vi "Keypad Facade.vi"(0 "Data In":T4, 2 "Display State In":T2, 3 "Container State":T3) -> (6 "Data Out":T4, 7 "Display State Out":T2, 8 "Action":T1)   [LabVIEW 2012, in "Keypad.xctl"]
uses:
  Keypad.xctl
  Keypad Data.ctl
  <vilib>/_xctls/Container State.ctl
  Keypad State.ctl
  <vilib>/_xctls/Action.ctl
  <vilib>/_xctls/XControlSupport.lvlib
panel:
  in  "C":bool
  in  "0":bool
  in  "E":bool
  in  "7":bool
  in  "8":bool
  in  "9":bool
  in  "4":bool
  in  "5":bool
  in  "6":bool
  in  "3":bool
  in  "2":bool
  in  "1":bool
  in  "Display":string
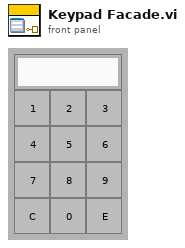
[diagram p1: front panel]
types:
  T1 = typedef "XControlSupport.lvlib/Action.ctl" = cluster{"Data Changed?":bool, "State Changed?":bool, "Action Name":string}
  T2 = typedef "Keypad.xctl/Keypad State.ctl" = cluster{"Current Value":i32}
  T3 = typedef "XControlSupport.lvlib/Container State.ctl" = cluster{"Indicator?":bool, "Run Mode?":bool, " Refnum":refnum<vi>}
  T4 = typedef "Keypad.xctl/Keypad Data.ctl" = i32
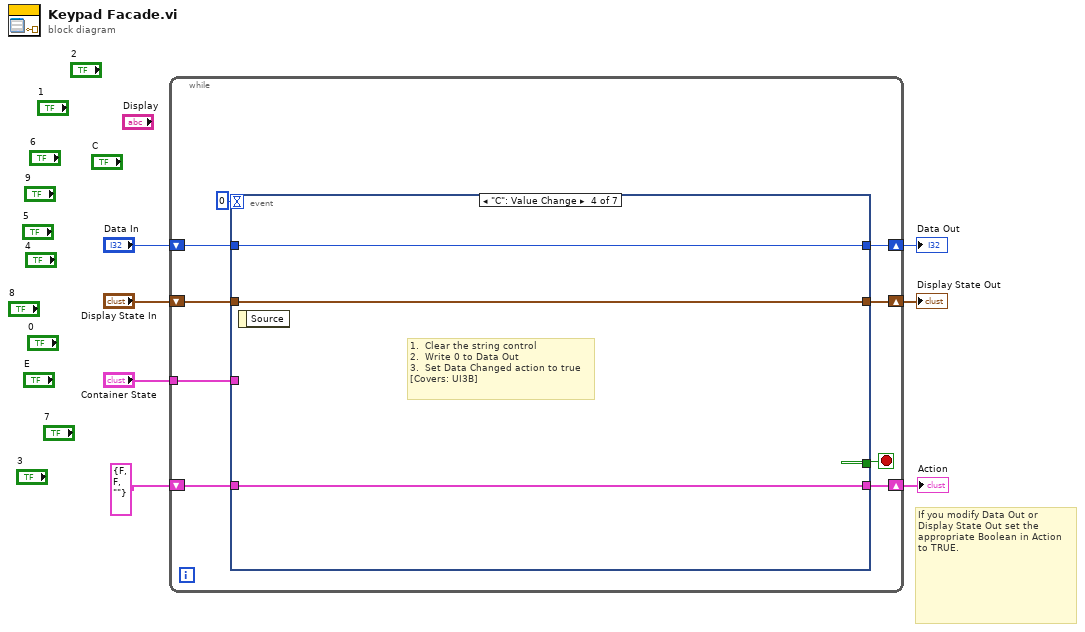
[diagram p0: block diagram]
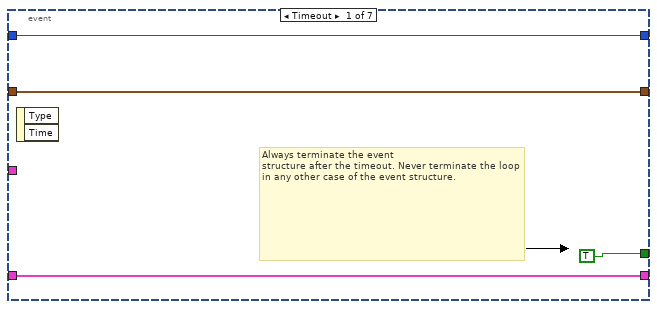
[diagram p2: hidden frame]
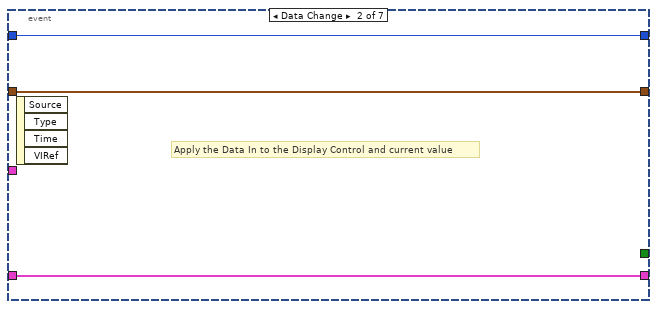
[diagram p3: hidden frame]
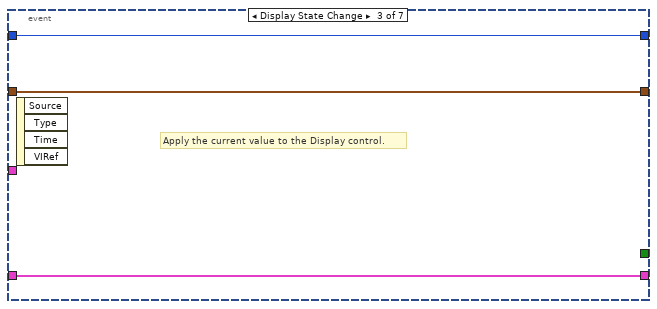
[diagram p4: hidden frame]
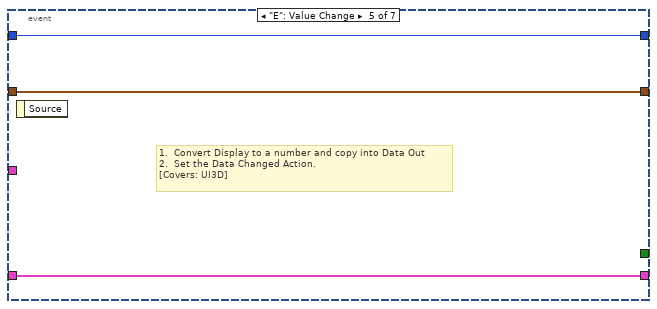
[diagram p5: hidden frame]
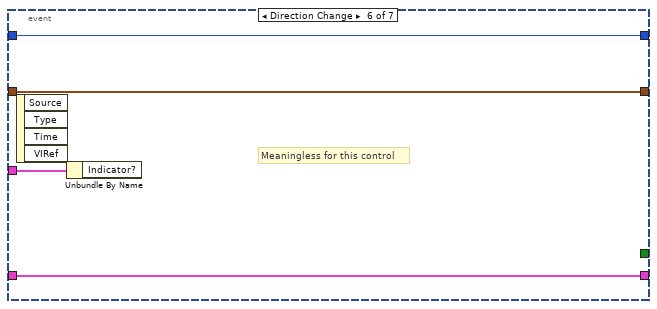
[diagram p6: hidden frame]
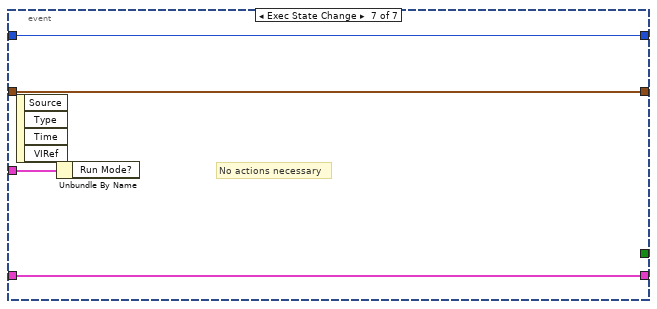
[diagram p7: hidden frame]
diagram:
  # "If you modify Data Out or\nDisplay State Out set the\nappropriate Boolean in Action\nto TRUE."
  n1 = while {
    shift-right: [w15] -> w4
    shift-left: "Display State In" -> [w16]
    tunnel: "Container State" -> [w12]
    shift-right: [w10] -> w7
    shift-left: "Data In" -> [w11]
    shift-right: [w8] -> w2
    shift-left: T1 {"Data Changed?"=FALSE, "State Changed?"=FALSE, "Action Name"=""} ("Action") -> [w9]
    stop <- w14 stop-if-true
    n2 = event shown="[3] \"C\": Value Change" {
      selector: _ -> [_ _ _ _ _ _ _]
      dyn-events: _ -> [_ _ _ _ _ _ _]
      timeout: 0 -> [_ _ _ _ _ _ _]
      tunnel: w16 -> [w18 w22 w26 w28 w31 w35 w39]
      tunnel: [w18 w22 w26 w28 w31 w35 w39] -> w15
      tunnel: [TRUE _ _ _ _ _ _] -> w14
      tunnel: w12 -> [_ _ _ _ _ w36 w40]
      tunnel: w11 -> [w17 w23 w25 w29 w32 w34 w38]
      tunnel: [w17 w23 w25 w29 w32 w34 w38] -> w10
      tunnel: [w19 w21 w24 w27 w30 w33 w37] -> w8
      tunnel: w9 -> [w19 w21 w24 w27 w30 w33 w37]
      event Timeout {
        # "Always terminate the event\nstructure after the timeout. Never terminate the loop in any other case of the event structure."
        n3 = event-data() -> ()  [unwired: 1 in, 2 out]
      }
      event Data Change {
        # "Apply the Data In to the Display Control and current value"
        n4 = event-data() -> ()  [unwired: 1 in, 4 out]
      }
      event Display State Change {
        # "Apply the current value to the Display control."
        n5 = event-data() -> ()  [unwired: 1 in, 4 out]
      }
      event "C": Value Change {
        # "1.  Clear the string control\n2.  Write 0 to Data Out\n3.  Set Data Changed action to true\n[Covers: UI3B]"
        n6 = event-data() -> ()  [unwired: 1 in, 1 out]
      }
      event "E": Value Change {
        # "1.  Convert Display to a number and copy into Data Out\n2.  Set the Data Changed Action.\n[Covers: UI3D]"
        n7 = event-data() -> ()  [unwired: 1 in, 1 out]
      }
      event Direction Change {
        # "Meaningless for this control"
        n8 = event-data() -> ()  [unwired: 1 in, 4 out]
        n9 = Unbundle By Name(w36) -> ()  [unwired: 1 out]
      }
      event Exec State Change {
        # "No actions necessary"
        n10 = event-data() -> ()  [unwired: 1 in, 4 out]
        n11 = Unbundle By Name(w40) -> ()  [unwired: 1 out]
      }
    }
  }
  "Display State Out" <- w4
  "Data Out" <- w7
  "Action" <- w2
